vi "GKC_Sayi_Secim_Ekrani.vi"() -> ()   [LabVIEW 2014]
uses:
  CustomControls/User_Selection.ctl
  CustomControls/Referans_Tip.ctl
  CustomControls/TSE_Status.ctl
  CustomControls/Program_States.ctl
panel:
  in  "Operatör":string="2" caption="Kalibrasyonu Yapan"
  in  "Cihazın Sahibi":string="TEİAŞ"
  in  "Ref Seri Numarası":string="1" caption="Seri Numarası"
  in  "Üretici":enum16{"", "FLUKE"}(ring)=enum."FLUKE"
  in  "Ref. Model":T1=enum."6105A" caption="Tip"
  out "?":string="Referans"
  in  "GKÇ Tip":enum16{"", "PQ+", "PQ++", "ION"}[](array[ring])=[enum."PQ++"] caption="Tip"
  in  "GKÇ Seri Numarası":string[](array[string])=["3", "", ""] caption="Seri Numarası"
  in  "Ölçüm Fonksiyonları":T2
  out "?":string="GKÇ 3"
  out "?":string="GKÇ 2"
  out "?":string="GKÇ 1"
  in  "Cancel Button":bool
  in  "OK Button":bool
  in  "IP Adresi":string[](array[string])=["", "", ""]
  in  "Üretici":T3[](array[typedef])=[enum."TÜBİTAK EE", enum."", enum.""]
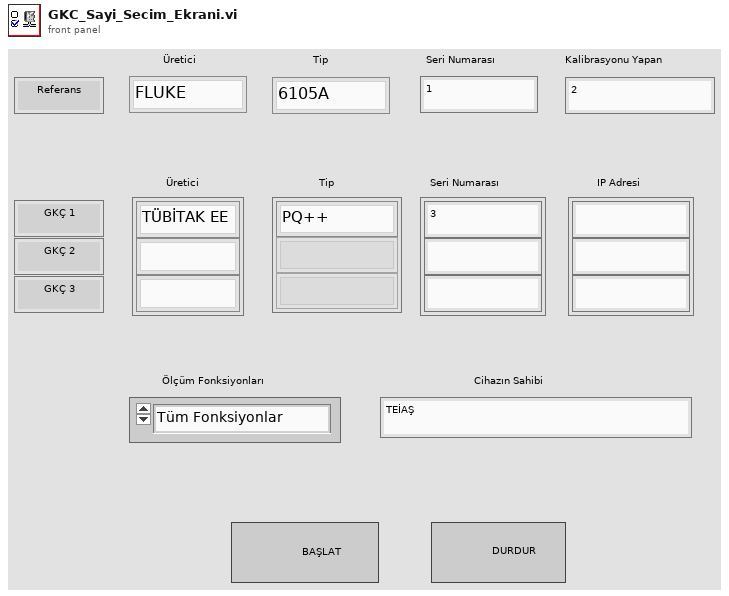
[diagram p1: front panel]
types:
  T1 = typedef "Referans_Tip.ctl" = enum16{"", "6105A"}
  T2 = typedef "User_Selection.ctl" = enum16{"Tüm Fonksiyonlar", "Frekans", "AC Gerilim", "AC Akım", "Aktif Güç", "Reaktif Güç", "Harmonik Akım", "Harmonik Gerilim", "Flicker", "Sertifika Oluştur"}
  T3 = typedef "GKÇ_Uretici.ctl" = enum16{"", "TÜBİTAK EE", "SCHNEIDER"}
  T4 = typedef "TSE_Status.ctl" = cluster{"Return Code":i32, "Message":string, "error in (no error)":errorcluster, "Program State":T5, "Test A. Suresi":u32}
  T5 = typedef "Program_States.ctl" = enum16{"Ön Yükleme", "TSE Baslat", "Kalibratöre Baglan", "Kalibratörü Baslat", "Ön Yükleme Tamam", "Frekans Testi", "Gerilim Testi", "Akim Testi", "Aktif Guc Testi", "Reaktif Guc Testi", "AC Akim Harmonik Testi", "AC Gerilim Harmonik Testi", "Flicker Testi", "Rapor Cikarma", "Yeniden Başlat", "Bekleme", "Durdur"}
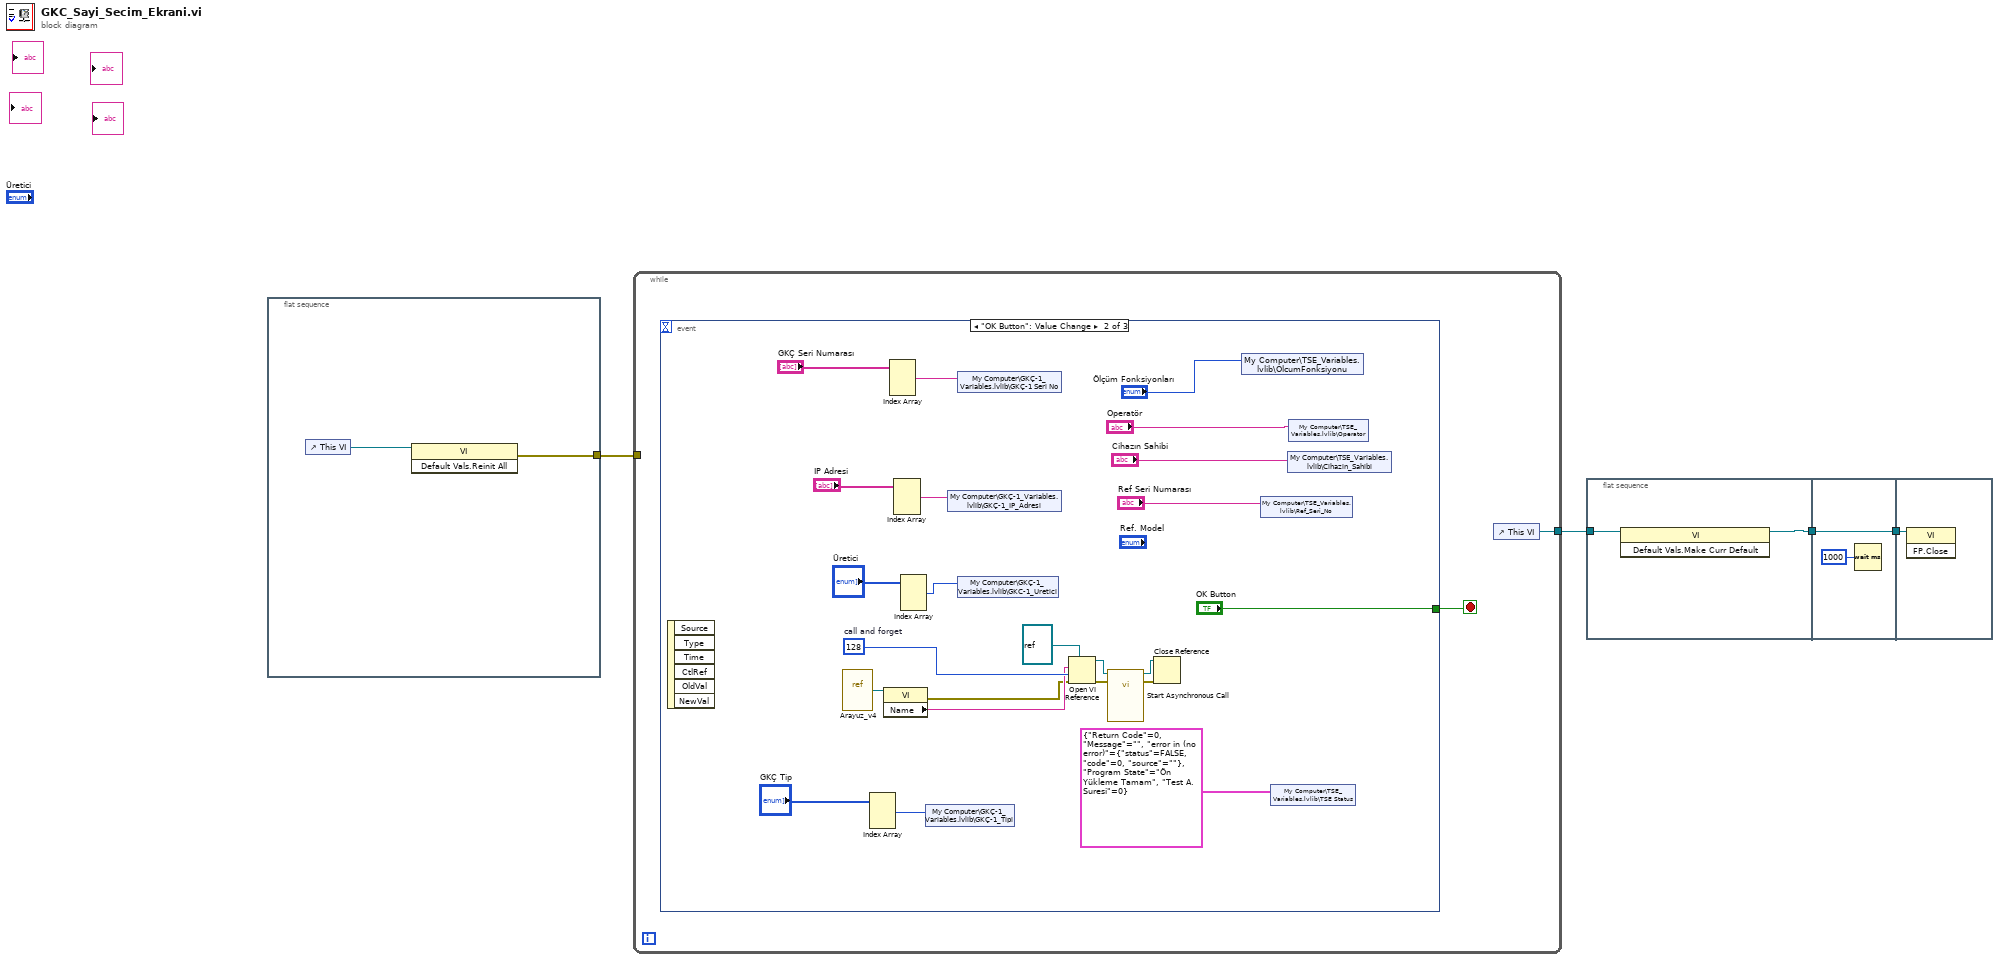
[diagram p0: block diagram]
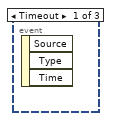
[diagram p2: hidden frame]
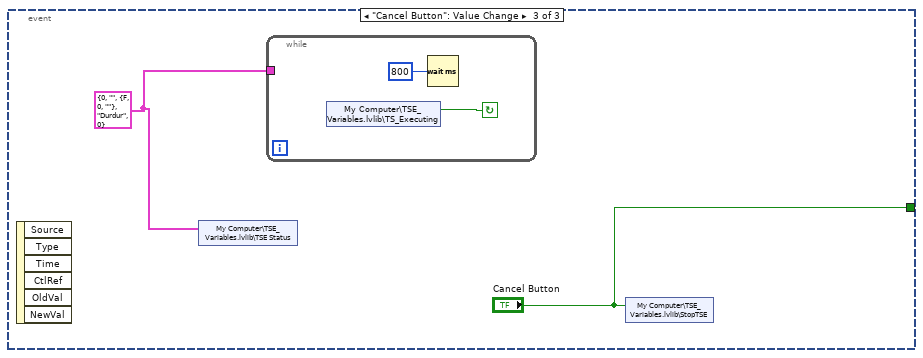
[diagram p3: hidden frame]
diagram:
  n1 = flat-sequence {
    tunnel: [w5] -> w2
    frame #0 {
      n2 = control-ref of="This VI"() -> (w6:refnum<vi>)
      n3 = invoke class="VI" method="Default Vals.Reinit All"(reference=w6) -> (error out=w5:errorcluster)  [unwired: 2 in, 2 out]
    }
  }
  n4 = while {
    tunnel: [w8] -> w4
    tunnel: w2 -> [_]
    stop <- w7 stop-if-true
    n5 = event shown="[1] \"OK Button\": Value Change" {
      selector: _ -> [_ _ _]
      dyn-events: _ -> [_ _ _]
      timeout: _ -> [_ _ _]
      tunnel: [_ "OK Button" "Cancel Button"] -> w7
      event Timeout {
        n6 = event-data() -> ()  [unwired: 1 in, 3 out]
      }
      event "OK Button": Value Change {
        w28 = 128  # call and forget
        n7 = event-data() -> ()  [unwired: 1 in, 6 out]
        n8 = vi-ref "Arayuz_v4.vi"() -> (w24:refnum<vi>)
        n9 = Index Array(array="GKÇ Tip") -> (element #1=w10:enum16{"", "PQ+", "PQ++", "ION"})  [unwired: 3 in, 2 out]
        n10 = property class="VI"(reference=w24) -> (error out=w22:errorcluster, "Name"=w23:string)  [unwired: 1 in, 1 out]
        n11 = Index Array(array="GKÇ Seri Numarası") -> (element #1=w13:string)  [unwired: 3 in, 2 out]
        n12 = Index Array(array="IP Adresi") -> (element #1=w12:string)  [unwired: 3 in, 2 out]
        n13 = Index Array(array="Üretici") -> (element #1=w9:T3)  [unwired: 3 in, 2 out]
        n14 = shared-variable "My Computer\\GKÇ-1_Variables.lvlib\\GKÇ-1_Tipi"(w10) -> ()  [unwired: 1 in, 1 out]
        n15 = shared-variable "My Computer\\GKÇ-1_Variables.lvlib\\GKÇ-1_IP_Adresi"(w12) -> ()  [unwired: 1 in, 1 out]
        n16 = shared-variable "My Computer\\GKÇ-1_Variables.lvlib\\GKC-1_Uretici"(w9) -> ()  [unwired: 1 in, 1 out]
        n17 = shared-variable "My Computer\\GKÇ-1_Variables.lvlib\\GKÇ-1 Seri No"(w13) -> ()  [unwired: 1 in, 1 out]
        n18 = Open VI Reference(type specifier VI Refnum (for type only)=refnum<vi> refnum, vi path=w23, options=w28, error in (no error)=w22) -> (vi reference=w21:refnum<vi>, error out=w27:errorcluster)  [unwired: 2 in]
        n19 = call-by-ref "Start Asynchronous Call"(reference=w21, error in=w27) -> (reference out=w25:refnum<vi>, error out=w26:errorcluster)  [unwired: 12 in]
        n20 = Close Reference(reference=w25, error in (no error)=w26) -> ()  [unwired: 1 out]
        n21 = shared-variable "My Computer\\TSE_Variables.lvlib\\OlcumFonksiyonu"("Ölçüm Fonksiyonları") -> ()  [unwired: 1 in, 1 out]
        n22 = shared-variable "My Computer\\TSE_Variables.lvlib\\Ref_Seri_No"("Ref Seri Numarası") -> ()  [unwired: 1 in, 1 out]
        n23 = shared-variable "My Computer\\TSE_Variables.lvlib\\TSE Status"(T4 {"Return Code"=0, "Message"="", "error in (no error)"={"status"=FALSE, "code"=0, "source"=""}, "Program State"=enum."Ön Yükleme Tamam", "Test A. Suresi"=0} ("TSE Status")) -> ()  [unwired: 1 in, 1 out]
        n24 = shared-variable "My Computer\\TSE_Variables.lvlib\\Cihazin_Sahibi"("Cihazın Sahibi") -> ()  [unwired: 1 in, 1 out]
        n25 = shared-variable "My Computer\\TSE_Variables.lvlib\\Operator"("Operatör") -> ()  [unwired: 1 in, 1 out]
      }
      event "Cancel Button": Value Change {
        w32 = T4 {"Return Code"=0, "Message"="", "error in (no error)"={"status"=FALSE, "code"=0, "source"=""}, "Program State"=enum."Durdur", "Test A. Suresi"=0} ("TSE Status")
        n26 = event-data() -> ()  [unwired: 1 in, 6 out]
        n27 = shared-variable "My Computer\\TSE_Variables.lvlib\\TSE Status"(w32) -> ()  [unwired: 1 in, 1 out]
        n28 = while {
          tunnel: w32 -> [_]
          stop <- w34 continue-if-true
          n29 = shared-variable "My Computer\\TSE_Variables.lvlib\\TS_Executing"() -> (w34:bool)  [unwired: 1 in, 1 out]
          n30 = Wait (ms)(milliseconds to wait=u32 800) -> ()  [unwired: 1 out]
        }
        n31 = shared-variable "My Computer\\TSE_Variables.lvlib\\StopTSE"("Cancel Button") -> ()  [unwired: 1 in, 1 out]
      }
    }
    n32 = control-ref of="This VI"() -> (w8:refnum<vi>)
  }
  n33 = flat-sequence {
    tunnel: w4 -> [w37]
    tunnel: [w36] -> w1
    tunnel: [w39] -> w3
    tunnel: w1 -> [w39]
    tunnel: w3 -> [w40]
    frame #0 {
      n34 = invoke class="VI" method="Default Vals.Make Curr Default"(reference=w37) -> (reference out=w36:refnum<vi>)  [unwired: 2 in, 2 out]
    }
    frame #1 {
      n35 = Wait (ms)(milliseconds to wait=u32 1000) -> ()  [unwired: 1 out]
    }
    frame #2 {
      n36 = invoke class="VI" method="FP.Close"(reference=w40) -> ()  [unwired: 2 in, 3 out]
    }
  }
